vi "Pre Launch Init.vi"(11 "Server in":refnum<class "Server.lvclass">) -> (0 "error out":errorcluster, 3 "Server out":refnum<class "Server.lvclass">)   [LabVIEW 2018, in "Server.lvlib" / "Server.lvclass"]
doc: "(<B>Filename</B>: Actor Framework.lvlib:Actor.lvclass:Pre Launch Init.vi)\n\nDefines behavior that occurs after the Launch Nested Actor method is invoked but before the actor's Actor Core method begins running.\n\nBy default, this method does nothing. A descendant class may override it to define behavior."
uses:
  Server.lvclass
  Server.lvclass/Server.ctl
  <vilib>/ActorFramework/Actor/Actor.lvclass
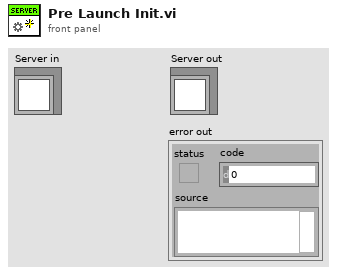
[diagram p1: front panel]
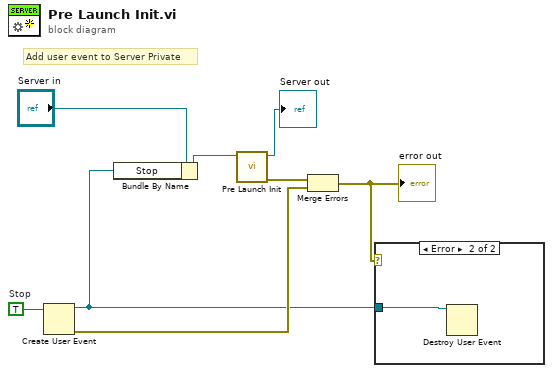
[diagram p0: block diagram]
diagram:
  w5 = TRUE  # Stop
  # "Add user event to Server Private"
  n1 = Create User Event(user event datatype=w5) -> (user event=w1:refnum<user-event>, error out=w3:errorcluster)  [unwired: 1 in]
  n2 = Bundle By Name(cluster="Server in", "Stop"=w1) -> (w4:refnum<class "Server.lvclass">)
  n3 = call-parent "Pre Launch Init.vi"("Actor in"=w4) -> ("error out"=w8:errorcluster, "Actor out"=→"Server out":refnum<class "Server.lvclass">)  [unwired: 9 in]
  n4 = Merge Errors(w8, w3) -> (w2:errorcluster)
  "error out" <- w2
  n5 = case shown="Error" w2 {
    tunnel: w1 -> [_ w9]
    frame No Error {
    }
    frame Error {
      n6 = Destroy User Event(user event=w9) -> ()  [unwired: 1 in, 1 out]
    }
  }
